vi "Start Scan.vi"(8 "error in (no error)":errorcluster, 9 "Scan Settings":T1, 10 "Model in":refnum<class "Model.lvclass">, 11 "Wait For User Input State in":refnum<class "Wait For User Input State.lvclass">) -> (0 "error out":errorcluster, 2 "Model out":refnum<class "Model.lvclass">, 3 "Wait For User Input State out":refnum<class "Wait For User Input State.lvclass">)   [LabVIEW 2015, in "Wait For User Input State.lvclass"]
uses:
  Wait For User Input State.lvclass
  Model/Model/Model.lvclass
  Typedefs/StateTypes.ctl
  Typedefs/FAMT Typedefs.lvlib
  Typedefs/ScanSettings.ctl
  Typedefs/WaveformTypes.ctl
  Typedefs/WaveformSettings.ctl
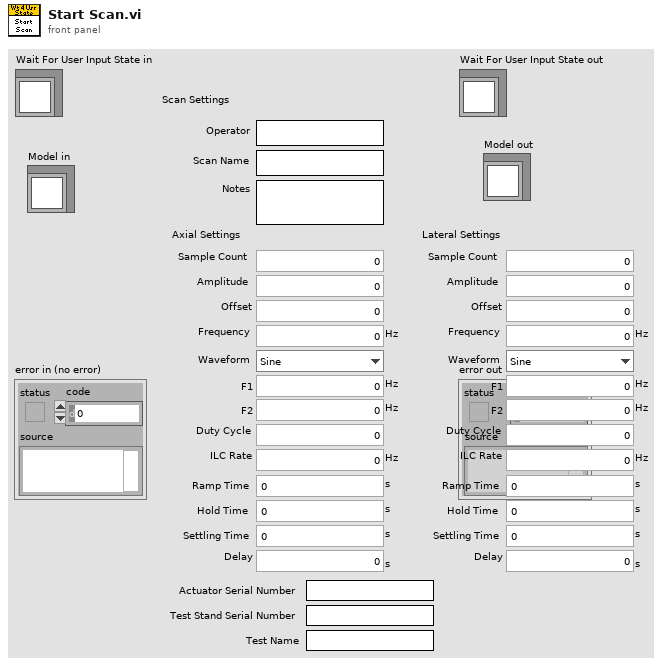
[diagram p1: front panel]
types:
  T1 = typedef "FAMT Typedefs.lvlib/ScanSettings.ctl" = cluster{"Operator":string, "Scan Name":string, "Notes":string, "Axial Settings":T2, "Lateral Settings":T2, "Actuator Serial Number":string, "Test Stand Serial Number":string, "Test Name":string}
  T2 = typedef "FAMT Typedefs.lvlib/WaveformSettings.ctl" = cluster{"Sample Count":u32, "Amplitude":dbl, "Offset":dbl, "Frequency":dbl[unit], "Waveform":T3, "F1":dbl[unit], "F2":dbl[unit], "Duty Cycle":dbl, "ILC Rate":dbl[unit], "Ramp Time":dbl[unit], "Hold Time":dbl[unit], "Settling Time":dbl[unit], "Delay":dbl[unit]}
  T3 = typedef "FAMT Typedefs.lvlib/WaveformTypes.ctl" = enum16{"Sine", "Triangle", "Square", "Sawtooth", "Chirp", "Gaussian", "Trapezoid", "Constant"}
  T4 = typedef "FAMT Typedefs.lvlib/StateTypes.ctl" = enum16{"Offline State", "Fault State", "Standby State", "Disabled State", "Enabled State", "Wait For User Input State", "Perform Scan State"}
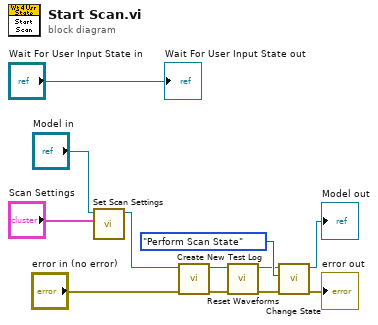
[diagram p0: block diagram]
diagram:
  n1 = call "Set Scan Settings.vi"("Scan Settings"="Scan Settings", "Model in"="Model in") -> ("Model out"=w1:refnum<class "Model.lvclass">)  [unwired: 9 in]
  n2 = call "Create New Test Log.vi"("error in (no error)"="error in (no error)", "Model in"=w1) -> ("error out"=w4:errorcluster, "Model out"=w3:refnum<class "Model.lvclass">)  [unwired: 8 in]
  n3 = call "Reset Waveforms.vi"("error in (no error)"=w4, "Model in"=w3) -> ("error out"=w6:errorcluster, "Model out"=w5:refnum<class "Model.lvclass">)  [unwired: 8 in]
  n4 = call "Change State.vi"("error in (no error)"=w6, "State Types"=StateTypes."Perform Scan State" ("State:"), "Model in"=w5) -> ("error out"=→"error out":errorcluster, "Model out"=→"Model out":refnum<class "Model.lvclass">)  [unwired: 7 in]
  "Wait For User Input State out" <- "Wait For User Input State in"
